vi "Assign Timing.vi"(8 "error in (no error)":errorcluster, 11 "Chassis Tasks in":refnum<class "Chassis Tasks.lvclass">) -> (0 "error out":errorcluster, 3 "Chassis Tasks out":refnum<class "Chassis Tasks.lvclass">)   [LabVIEW 2018, in "Data Acquisition.lvlib" / "Chassis Tasks.lvclass"]
uses:
  Chassis Tasks.lvclass
  Chassis Tasks.lvclass/Chassis Tasks.ctl
  Class DAQ Task/DAQ Task.lvclass
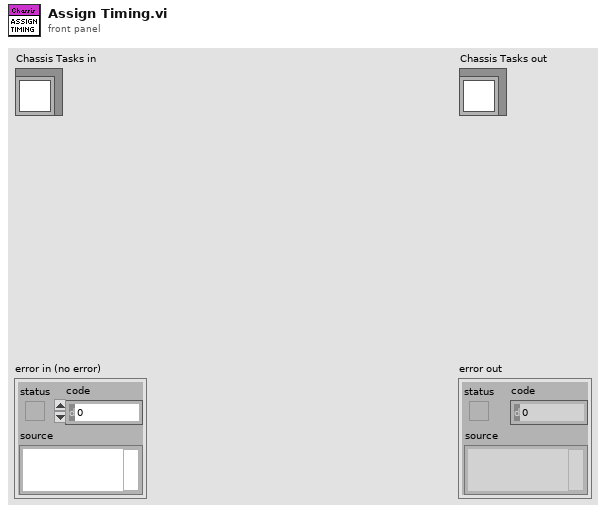
[diagram p1: front panel]
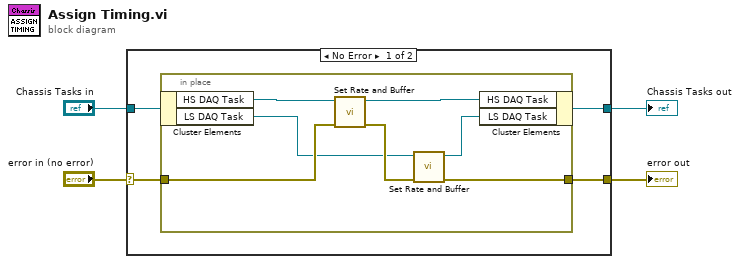
[diagram p0: block diagram]
diagram:
  n1 = case shown="No Error" "error in (no error)" {
    selector: "error in (no error)" -> [w7 w17]
    tunnel: [w6 w17] -> w3
    tunnel: [w5 w16] -> w1
    tunnel: "Chassis Tasks in" -> [w8 w16]
    frame No Error {
      n2 = in-place {
        in-place-border: w7 -> [w14]
        in-place-border: [w12] -> w6
        n3 = in-place-cluster #1(w8) -> ("HS DAQ Task"=w15:refnum<class "DAQ Task.lvclass">, "LS DAQ Task"=w10:refnum<class "DAQ Task.lvclass">)
        n4 = call "Set Rate and Buffer.vi"("error in (no error)"=w14, "DAQ Task in"=w15) -> ("error out"=w13:errorcluster, "DAQ Task out"=w11:refnum<class "DAQ Task.lvclass">)  [unwired: 8 in]
        n5 = call "Set Rate and Buffer.vi"("error in (no error)"=w13, "DAQ Task in"=w10) -> ("error out"=w12:errorcluster, "DAQ Task out"=w9:refnum<class "DAQ Task.lvclass">)  [unwired: 8 in]
        n6 = in-place-cluster #1("HS DAQ Task"=w11, "LS DAQ Task"=w9) -> (w5:refnum<class "Chassis Tasks.lvclass">)
      }
    }
    frame Error {
    }
  }
  "error out" <- w3
  "Chassis Tasks out" <- w1
